vi "Analyzer.GetRequirement_FGV.vi"(7 "Operation":enum16{"Reset", "Get"}(ring), 8 "error in":errorcluster, 10 "List of Words":string[](array[string])) -> (0 "error out":errorcluster, 1 "Empty Word":bool, 2 "Word for search":string)   [LabVIEW 2022 SP3, in "Analyzer.lvclass"]
uses:
  Analyzer.lvclass
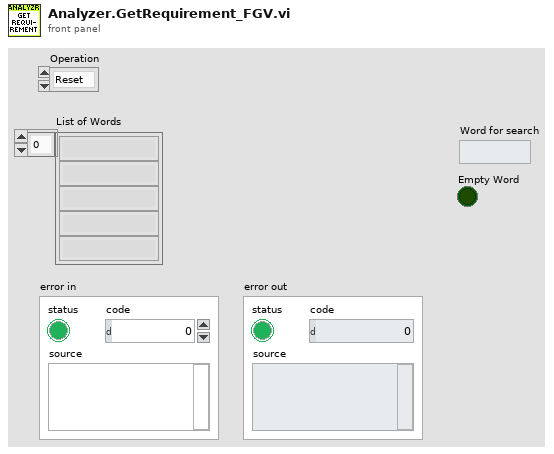
[diagram p1: front panel]
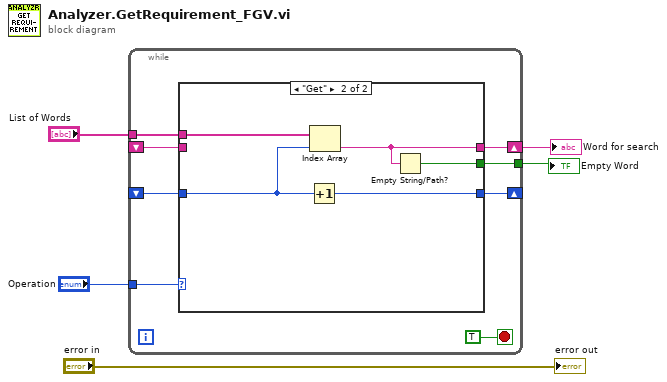
[diagram p0: block diagram]
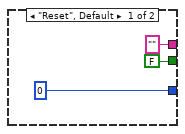
[diagram p2: hidden frame]
diagram:
  n1 = while {
    tunnel: "Operation" -> [w13]
    shift-right: [w12] -> _
    shift-left: _ -> [w9]
    tunnel: "List of Words" -> [w11]
    shift-right: [w8] -> w3
    shift-left: _ -> [w7]
    tunnel: [w6] -> w2
    stop <- TRUE stop-if-true
    n2 = case shown="\"Get\"" w13 {
      tunnel: [0 w19] -> w12
      tunnel: w11 -> [_ w21]
      tunnel: w9 -> [_ w20]
      tunnel: ["" ("String") w18] -> w8
      tunnel: w7 -> [_ _]
      tunnel: [FALSE w17] -> w6
      frame "Reset", Default {
      }
      frame "Get" {
        n3 = Increment(x=w20) -> (x+1=w19:i32)
        n4 = Index Array(array=w21, index=w20) -> (element=w18:string)
        n5 = Empty String/Path?(string/path=w18) -> (empty?=w17:bool)
      }
    }
  }
  "Word for search" <- w3
  "Empty Word" <- w2
  "error out" <- "error in"
